vi "电子1691余志凯201641053015.vi"(1 "b":dbl, 2 "x":dbl, 3 "k":dbl) -> (0 "y":dbl)   [LabVIEW 2017]
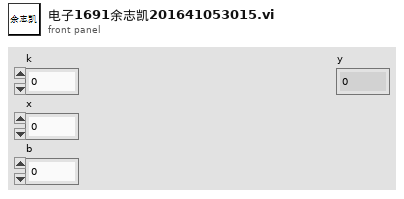
[diagram p1: front panel]
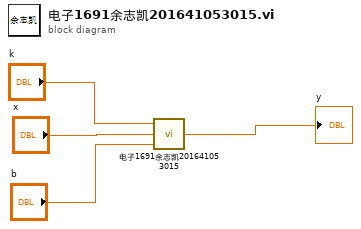
[diagram p0: block diagram]
diagram:
  n1 = call "电子1691余志凯201641053015.vi"("b"="b", "x"="x", "k"="k") -> ("y"=→"y":dbl)
